vi "temperature.vi"() -> ()   [LabVIEW 2012]
uses:
  <vilib>/Analysis/5stat.llb/RMS (DBL).vi
  <vilib>/Analysis/NI_AALPro.lvlib
panel:
  in  "Sound":bool
  out "Low\n temp!":bool
  out "Mouse \nTemp":dbl(slide) scale=30.0..40.0
  in  "stop (F)":bool
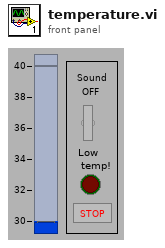
[diagram p1: front panel]
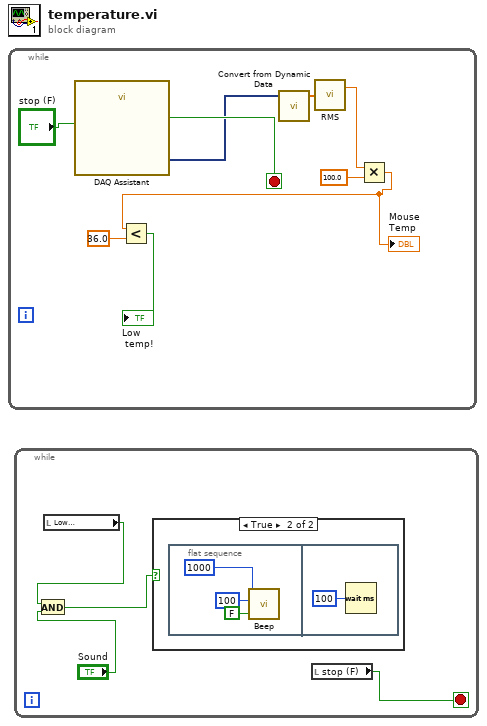
[diagram p0: block diagram]
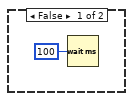
[diagram p2: hidden frame]
diagram:
  n1 = while {
    stop <- w8 stop-if-true
    n2 = call "DAQ Assistant"("stop (F)"="stop (F)") -> ("data"=w6:dynamicdata, "stopped"=w8:bool)  [unwired: 15 in, 2 out]
    n3 = call "Convert from Dynamic Data"("Dynamic Data Type"=w6) -> ("Array"=w7:dbl[])  [unwired: 3 in]
    n4 = call-poly <vilib>:"RMS.vi"("X"=w7) -> ("rms value"=w4:dbl)  [unwired: 1 out]
    n5 = Multiply(x=w4, y=100.0) -> (x*y=w2:dbl)
    "Mouse \nTemp" <- w2
    n6 = Less?(x=w2, y=36.0) -> (x < y?=→"Low\n temp!":bool)
  }
  n7 = while {
    stop <- w13 stop-if-true
    n8 = local read "Low\n temp!"() -> (w12:bool)
    n9 = And(x=w12, y="Sound") -> (x .and. y?=w10:bool)
    n10 = case shown="True" w10 {
      frame False {
        n11 = Wait (ms)(milliseconds to wait=u32 100) -> ()  [unwired: 1 out]
      }
      frame True {
        n12 = flat-sequence {
          frame #0 {
            n13 = call <vilib>:"Beep.vi"("use system alert? (T)"=FALSE, "duration (msec)"=u32 100, "frequency (Hz)"=u32 1000) -> ()  [unwired: 9 in]
          }
          frame #1 {
            n14 = Wait (ms)(milliseconds to wait=u32 100) -> ()  [unwired: 1 out]
          }
        }
      }
    }
    n15 = local read "stop (F)"() -> (w13:bool)
  }
